vi "Get Core Type.vi"(8 "error in (no error)":errorcluster, 11 "Sequencer in":refnum<class "Sequencer.lvclass">) -> (0 "error out":errorcluster, 3 "Sequencer Core out":refnum<class "Sequencer Core.lvclass">)   [LabVIEW 2020, in "Sequencer.lvlib" / "Sequencer.lvclass"]
doc: "Return the Sequencer Core type to launch with the Sequencer."
uses:
  Sequencer.lvclass
  Sequencer Core/Sequencer Core.lvclass
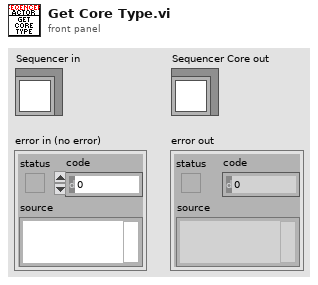
[diagram p1: front panel]
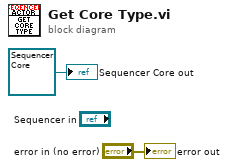
[diagram p0: block diagram]
diagram:
  "error out" <- "error in (no error)"
  "Sequencer Core out" <- refnum<class "Sequencer Core.lvclass"> refnum ("Sequencer Core out")
